vi "Read Recipe Data Save Location.vi"(8 "error in (no error)":errorcluster, 11 "Recipe State Data in":refnum<class "Recipe State Data.lvclass">) -> (0 "error out":errorcluster, 2 "Recipe Data Save Location":path, 3 "Recipe State Data out":refnum<class "Recipe State Data.lvclass">)   [LabVIEW 2022 SP3, in "Recipe State Data.lvclass"]
uses:
  Recipe State Data.lvclass
  Recipe State Data.lvclass/Recipe State Data.ctl
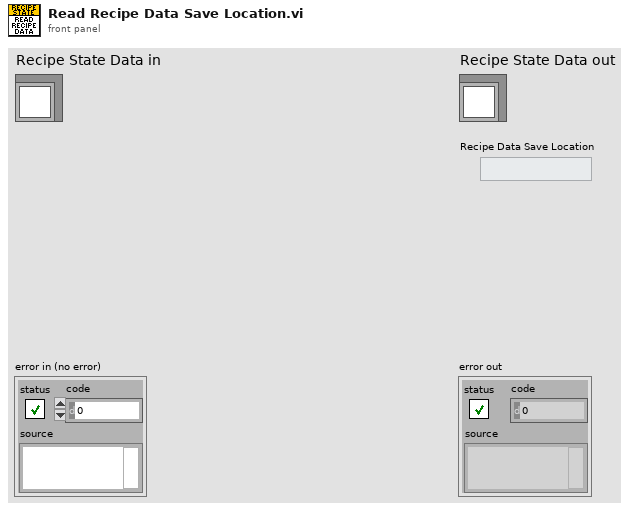
[diagram p1: front panel]
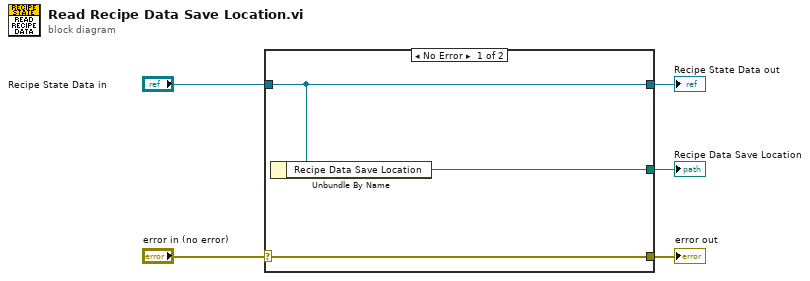
[diagram p0: block diagram]
diagram:
  n1 = case shown="No Error" "error in (no error)" {
    selector: "error in (no error)" -> [w8 w9]
    tunnel: [w8 w9] -> w4
    tunnel: [w7 w10] -> w2
    tunnel: "Recipe State Data in" -> [w7 w10]
    tunnel: [w6 _] -> w1
    frame No Error {
      n2 = Unbundle By Name(w7) -> ("Recipe Data Save Location"=w6:path)
    }
    frame Error {
    }
  }
  "error out" <- w4
  "Recipe State Data out" <- w2
  "Recipe Data Save Location" <- w1
